vi "VI Tree.vi"   [LabVIEW 2016]
uses:
  Modules/DAQ-Display/PCM PanelSplit/SubClass/PCM MenuVIPanelSplit.lvclass
  Modules/DAQ-Display/PCM PanelSplit/PCM PanelSplit.lvclass
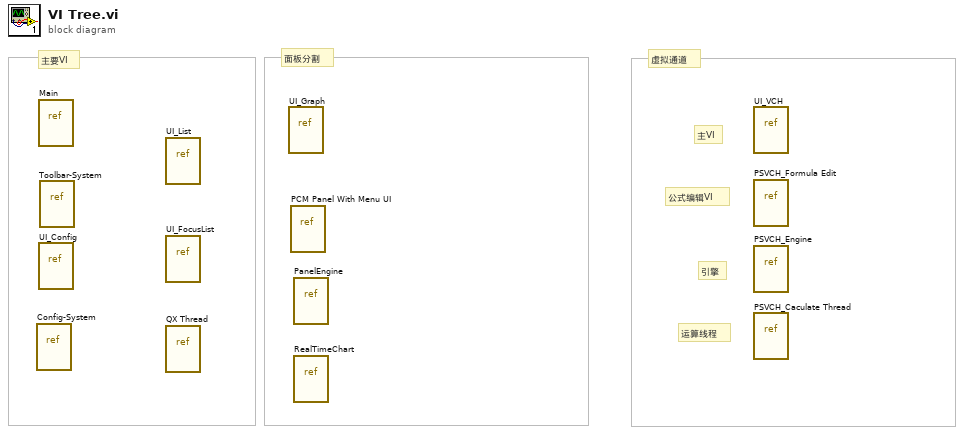
[diagram p0: block diagram]
diagram:
  # "主要VI"
  # "面板分割"
  # "虚拟通道"
  # "运算线程"
  # "引擎"
  # "公式编辑VI"
  # "主VI"
  n1 = vi-ref "Config-System.vi"() -> ()  [unwired: 1 out]
  n2 = vi-ref "Main.vi"() -> ()  [unwired: 1 out]
  n3 = vi-ref "UI_Config.vi"() -> ()  [unwired: 1 out]
  n4 = vi-ref "Toolbar-System.vi"() -> ()  [unwired: 1 out]
  n5 = vi-ref "UI_List.vi"() -> ()  [unwired: 1 out]
  n6 = vi-ref "UI_FocusList.vi"() -> ()  [unwired: 1 out]
  n7 = vi-ref "QX Thread.vi"() -> ()  [unwired: 1 out]
  n8 = vi-ref "UI_Graph.vi"() -> ()  [unwired: 1 out]
  n9 = vi-ref "PCM Panel With Menu UI.vi"() -> ()  [unwired: 1 out]
  n10 = vi-ref "PanelEngine.vi"() -> ()  [unwired: 1 out]
  n11 = vi-ref "RealTimeChart.vi"() -> ()  [unwired: 1 out]
  n12 = vi-ref "UI_VCH.vi"() -> ()  [unwired: 1 out]
  n13 = vi-ref "PSVCH_Formula Edit.vi"() -> ()  [unwired: 1 out]
  n14 = vi-ref "PSVCH_Engine.vi"() -> ()  [unwired: 1 out]
  n15 = vi-ref "PSVCH_Caculate Thread.vi"() -> ()  [unwired: 1 out]
